vi "Confirm Button.vi"(9 "reset":bool, 11 "Button":bool) -> (3 "Boolean out":bool)   [LabVIEW 2015]
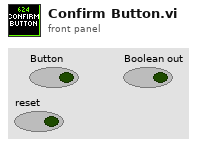
[diagram p1: front panel]
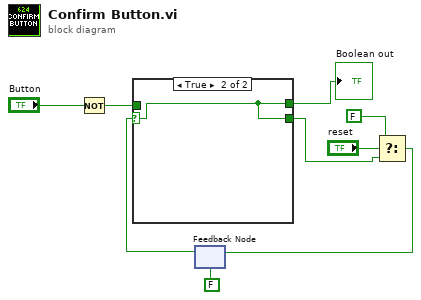
[diagram p0: block diagram]
diagram:
  n1 = Not(x="Button") -> (.not. x?=w8:bool)
  n2 = feedback #1(FALSE) -> (w7:bool)
  n3 = case shown="True" w7 {
    selector: w7 -> [_ w11]
    tunnel: [w10 w11] -> w3
    tunnel: [_ w11] -> w6
    tunnel: w8 -> [w10 _]
    frame False {
    }
    frame True {
    }
  }
  "Boolean out" <- w6
  n4 = Select(t=FALSE, s="reset", f=w3) -> (s? t:f=w1:bool)
  n5 = feedback-in #1(w1) -> ()
